vi "Configure Trigger (Edge).vi"(0 "VISA resource name":refnum<visa-resource-name>, 1 "Coupling (0:DC)":u16(ring) items=["DC", "AC", "Hf Reject", "Lf Reject", "Noise Rej", "Atrigger"], 2 "Trigger Event (0:A Event)":u16(ring) items=["A Event", "B Event"], 5 "Source (0:Channel1)":u16(ring) items=["Channel1"=0, "Channel2"=1, "Channel3"=2, "Channel4"=3, "Aux"=12, "Line"=13, "Digital Channel0"=14, "Digital Channel1"=15, "Digital Channel2"=16, "Digital Channel3"=17, "Digital Channel4"=18, "Digital Chennel5"=19, "Digital Channel6"=20, "Digital Channel7"=21, "Digital Channel8"=22, "Digital Channel9"=23, "Digital Channel10"=24, "Digital Channel11"=25, "Digital Channel12"=26, "Digital Channel13"=27, "Digital Channel14"=28, "Digital Channel15"=29], 7 "Trigger Level (0.0V)":dbl, 9 "Slope (0:Rise)":u16(ring) items=["Rise", "Fall", "Either"], 11 "error in (no error)":errorcluster) -> (4 "VISA resource name out":refnum<visa-resource-name>, 15 "error out":errorcluster)   [LabVIEW 2015, in "Tektronix 7000 Series.lvlib"]
doc: "Configures edge trigger settings for an oscilloscope. An edge trigger occurs when the trigger signal passes through the voltage threshold that you specify in <B>Trigger Level</B> and has the slope that you specify in <B>Trigger Slope</B>."
uses:
  <instrlib>/Tektronix 7000 Series/Tektronix 7000 Series.lvlib
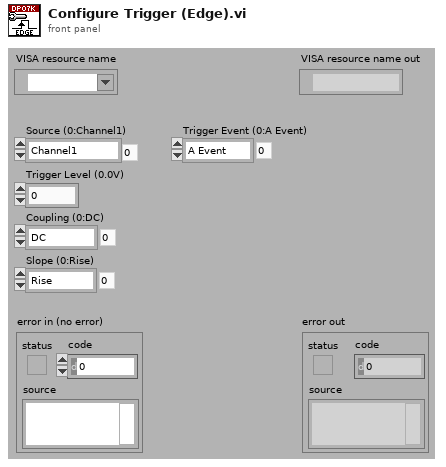
[diagram p1: front panel]
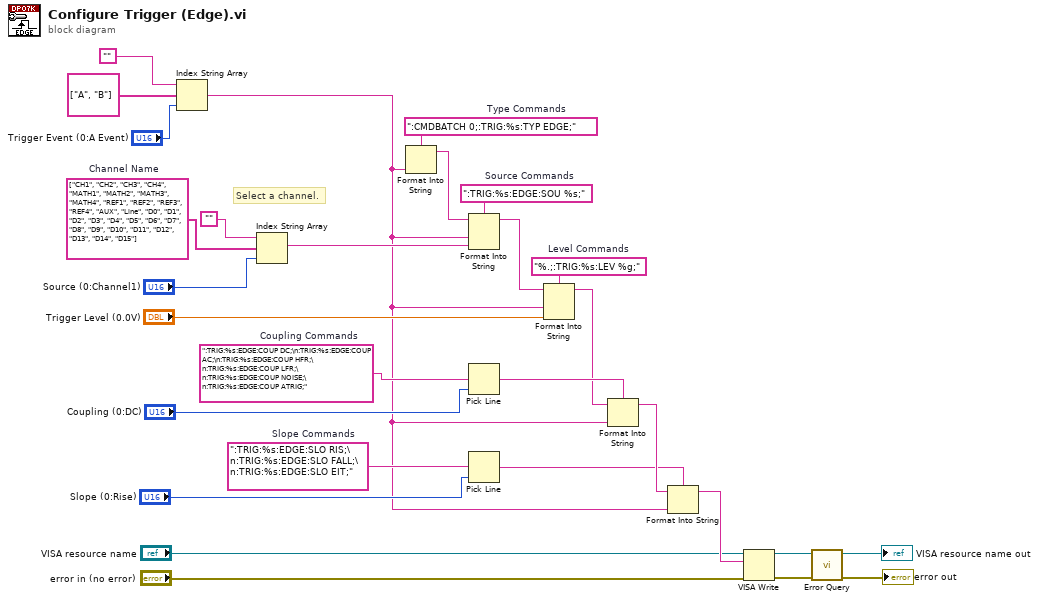
[diagram p0: block diagram]
diagram:
  w14 = ":TRIG:%s:EDGE:SLO RIS;\n:TRIG:%s:EDGE:SLO FALL;\n:TRIG:%s:EDGE:SLO EIT;"  # Slope Commands
  w15 = ":TRIG:%s:EDGE:COUP DC;\n:TRIG:%s:EDGE:COUP AC;\n:TRIG:%s:EDGE:COUP HFR;\n:TRIG:%s:EDGE:COUP LFR;\n:TRIG:%s:EDGE:COUP NOISE;\n:TRIG:%s:EDGE:COUP ATRIG;"  # Coupling Commands
  w16 = "%.;:TRIG:%s:LEV %g;"  # Level Commands
  w17 = ":TRIG:%s:EDGE:SOU %s;"  # Source Commands
  w11 = ":CMDBATCH 0;:TRIG:%s:TYP EDGE;"  # Type Commands
  w28 = string[] ["CH1", "CH2", "CH3", "CH4", "MATH1", "MATH2", "MATH3", "MATH4", "REF1", "REF2", "REF3", "REF4", "AUX", "Line", "D0", "D1", "D2", "D3", "D4", "D5", "D6", "D7", "D8", "D9", "D10", "D11", "D12", "D13", "D14", "D15"]  # Channel Name
  # "Select a channel."
  n1 = Index String Array(1:"Trigger Event (0:A Event)", 2:string[] ["A", "B"], 3:"" ("Empty String Constant")) -> (0:w4:string)
  n2 = Index String Array(1:"Source (0:Channel1)", 2:w28, 3:"" ("Empty String Constant")) -> (0:w12:string)
  n3 = Format Into String(format string=w11, w4) -> (resulting string=w10:string)  [unwired: 2 in, 1 out]
  n4 = Format Into String(format string=w17, initial string=w10, w4, w12) -> (resulting string=w13:string)  [unwired: 1 in, 1 out]
  n5 = Pick Line(multi-line string=w15, line index="Coupling (0:DC)") -> (output string=w8:string)  [unwired: 1 in]
  n6 = Pick Line(multi-line string=w14, line index="Slope (0:Rise)") -> (output string=w5:string)  [unwired: 1 in]
  n7 = Format Into String(format string=w16, initial string=w13, w4, "Trigger Level (0.0V)") -> (resulting string=w7:string)  [unwired: 1 in, 1 out]
  n8 = Format Into String(format string=w8, initial string=w7, w4) -> (resulting string=w6:string)  [unwired: 1 in, 1 out]
  n9 = Format Into String(format string=w5, initial string=w6, w4) -> (resulting string=w3:string)  [unwired: 1 in, 1 out]
  n10 = VISA Write(VISA resource name="VISA resource name", write buffer=w3, error in (no error)="error in (no error)") -> (VISA resource name out=w24:refnum<visa-resource-name>, error out=w25:errorcluster)  [unwired: 1 out]
  n11 = call <instrlib>:"Error Query.vi"("error in (no error)"=w25, "VISA resource name"=w24) -> ("error out"=→"error out":errorcluster, "VISA resource name out"=→"VISA resource name out":refnum<visa-resource-name>)  [unwired: 6 in, 2 out]
